vi "Force AR ALL.vi"(8 "error in (no error)":errorcluster, 11 "D&C_SchemaBase in":refnum<class "D&C_SchemaBase.lvclass">) -> (0 "error out":errorcluster, 3 "D&C_SchemaBase out":refnum<class "D&C_SchemaBase.lvclass">)   [LabVIEW 2020, in "D&C_SchemaBase.lvlib" / "D&C_SchemaBase.lvclass"]
uses:
  D&C_SchemaBase.lvclass
  support/UI_Actor.lvlibp/UI_Actor/ctl_AR_Mode.ctl
  support/UI_Actor.lvlibp/UI_Actor/UI_Actor.lvclass
  support/UI_Actor.lvlibp/UI_Actor/ctl_AR_Parameters.ctl
  support/Databox.lvlibp/TypesTools/Data/Data.lvclass
  support/Databox.lvlibp/TypesTools/Config/Config.lvclass
  D:/Projets/STEP AT/Bahamut/support/UI_Actor.lvlibp/UI_Actor/UI_Actor.lvclass
  D:/Projets/STEP AT/Bahamut/support/Actor Framework.lvlibp/1abvi3w/vi.lib/ActorFramework/Actor/Actor.lvclass
  D:/Projets/STEP AT/Bahamut/D&Cs/D&C_SchemaBase/D&C_SchemaBase/D&C_SchemaBase.lvclass
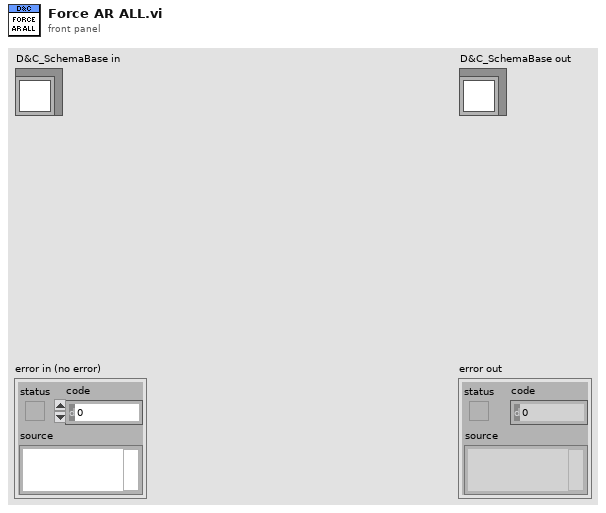
[diagram p1: front panel]
types:
  T1 = typedef "UI_Actor.lvlibp/UI_Actor.lvclass/ctl_AR_Parameters.ctl" = cluster{"Write TipStrips with details (T)":bool, "Write Captions with UserLabels (T)":bool, "Mode (ind only)":T2}
  T2 = typedef "UI_Actor.lvlibp/UI_Actor.lvclass/ctl_AR_Mode.ctl" = enum16{"Controls only", "Indicators only", "All"}
  T3 = cluster{"Ch.Conf":refnum<class "Config.lvclass">, "Data":refnum<class "Data.lvclass">[]}
  T4 = typedef "UI_Actor.lvlibp/UI_Actor.lvclass/ctl_InternalMapItem.ctl" = cluster{"Config":refnum<class "Config.lvclass">, "LatestData":refnum<class "Data.lvclass">}
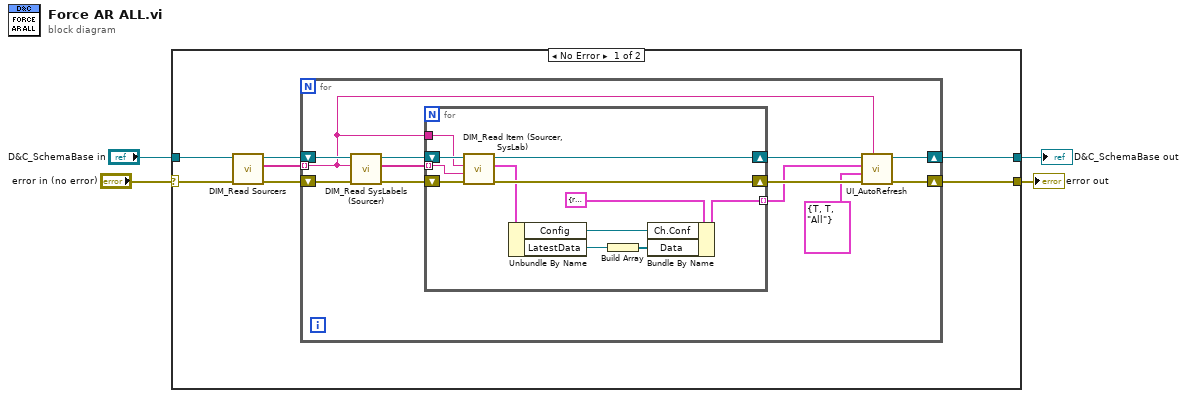
[diagram p0: block diagram]
diagram:
  n1 = case shown="No Error" "error in (no error)" {
    selector: "error in (no error)" -> [w8 w37]
    tunnel: [w7 w37] -> w3
    tunnel: [w6 w36] -> w1
    tunnel: "D&C_SchemaBase in" -> [w9 w36]
    frame No Error {
      n2 = call "DIM_Read Sourcers.vi"("error in (no error)"=w8, "UI_Actor in"=w9) -> ("error out"=w10:errorcluster, "DIM Sourcers"=w5:string[], "UI_Actor out"=w11:refnum<class "D&C_SchemaBase.lvclass">)  [unwired: 7 in]
      n3 = for {
        shift-right: [w16] -> w6
        shift-left: w11 -> [w23]
        shift-right: [w17] -> w7
        shift-left: w10 -> [w22]
        tunnel: w5 -> [w13] mode=indexing
        n4 = call "DIM_Read SysLabels (Sourcer).vi"("error in (no error)"=w22, "Sourcer"=w13, "UI_Actor in"=w23) -> ("error out"=w20:errorcluster, "DIM Sourcer's SysLabels"=w14:string[], "UI_Actor out"=w21:refnum<class "D&C_SchemaBase.lvclass">)  [unwired: 6 in]
        n5 = for {
          shift-right: [w33] -> w19
          shift-left: w21 -> [w35]
          shift-right: [w32] -> w18
          shift-left: w20 -> [w34]
          tunnel: w14 -> [w31] mode=indexing
          tunnel: w13 -> [w30]
          tunnel: [w27] -> w12 mode=indexing
          n6 = call "DIM_Read Item (Sourcer, SysLab).vi"("error in (no error)"=w34, "SysLabel"=w31, "Sourcer"=w30, "UI_Actor in"=w35) -> ("error out"=w32:errorcluster, "DIM Item"=w29:T4, "UI_Actor out"=w33:refnum<class "D&C_SchemaBase.lvclass">)  [unwired: 4 in, 1 out]
          n7 = Unbundle By Name(w29) -> ("Config"=w26:refnum<class "Config.lvclass">, "LatestData"=w25:refnum<class "Data.lvclass">)
          n8 = Build Array(w25) -> (w24:refnum<class "Data.lvclass">[])
          n9 = Bundle By Name(cluster=T3 {"Ch.Conf"=refnum, "Data"=[]} ("Cluster"), "Ch.Conf"=w26, "Data"=w24) -> (w27:T3)
        }
        n10 = call "UI_AutoRefresh.vi"("Sourcer name"=w13, "error in (no error)"=w18, "Parameters (Tipstrips,Captions,All)"=T1 {"Write TipStrips with details (T)"=TRUE, "Write Captions with UserLabels (T)"=TRUE, "Mode (ind only)"=enum."All"}, "Data chunk"=w12, "UI_Actor in"=w19) -> ("error out"=w17:errorcluster, "UI_Actor out"=w16:refnum<class "D&C_SchemaBase.lvclass">)  [unwired: 5 in]
      }
    }
    frame Error {
    }
  }
  "error out" <- w3
  "D&C_SchemaBase out" <- w1
